vi "VI, Set Window Position.vi"(4 "y (5)":i16=5, 5 "x (5)":i16=5, 6 "error in":errorcluster, 9 "VI ref":refnum<vi>) -> (0 "error out":errorcluster, 3 "VI ref dup":refnum<vi>)   [LabVIEW 2010]
doc: "This function sets the panel position in screen coordinates. The upper left outside corner of the panel is set to the x,y screen coordinate."
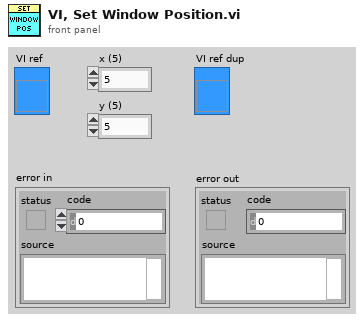
[diagram p1: front panel]
types:
  T1 = typedef "LVRectTypeDef.ctl" = cluster{"left":i16, "top":i16, "right":i16, "bottom":i16}
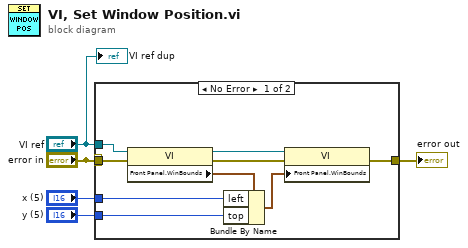
[diagram p0: block diagram]
diagram:
  n1 = case shown="No Error" "error in" {
    selector: "error in" -> [w14 w15]
    tunnel: [w11 w15] -> w5
    tunnel: "VI ref" -> [w13 _]
    tunnel: "error in" -> [_ _]
    tunnel: "x (5)" -> [w7 _]
    tunnel: "y (5)" -> [w6 _]
    frame No Error {
      n2 = property class="VI"(reference=w13, error in=w14) -> (reference out=w10:refnum<vi>, error out=w12:errorcluster, "Front Panel.WinBounds"=w9:T1)
      n3 = Bundle By Name(cluster=w9, "left"=w7, "top"=w6) -> (w8:T1)
      n4 = property class="VI"(reference=w10, error in=w12, "Front Panel.WinBounds"=w8) -> (error out=w11:errorcluster)  [unwired: 1 out]
    }
    frame Error {
    }
  }
  "error out" <- w5
  "VI ref dup" <- "VI ref"
